vi "Read Actual Values.vi"(8 "Error In":errorcluster, 11 "INL DNL Test in":refnum<class "INL DNL Test.lvclass">) -> (0 "Error Out":errorcluster, 2 "Actual Values":T1, 3 "INL DNL Test out":refnum<class "INL DNL Test.lvclass">)   [LabVIEW 2020, in "INL DNL Test.lvclass"]
uses:
  INL DNL Test.lvclass
  Device/Parent/Typedef/Data Cluster.ctl
  INL DNL Test.lvclass/INL DNL Test.ctl
  Device/Parent/Device.lvclass
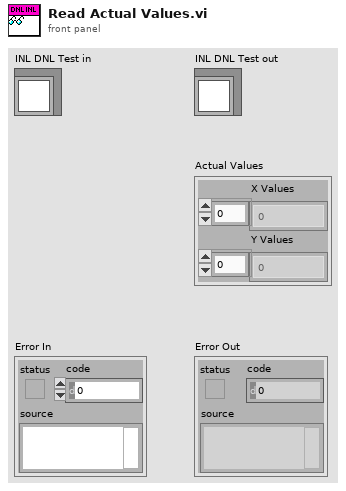
[diagram p1: front panel]
types:
  T1 = typedef "Device.lvclass/Data Cluster.ctl" = cluster{"X Values":dbl[], "Y Values":dbl[]}
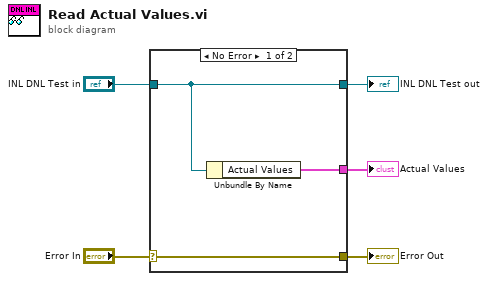
[diagram p0: block diagram]
diagram:
  n1 = case shown="No Error" "Error In" {
    selector: "Error In" -> [w8 w9]
    tunnel: [w8 w9] -> w4
    tunnel: [w7 w10] -> w2
    tunnel: "INL DNL Test in" -> [w7 w10]
    tunnel: [w6 _] -> w1
    frame No Error {
      n2 = Unbundle By Name(w7) -> ("Actual Values"=w6:T1)
    }
    frame Error {
    }
  }
  "Error Out" <- w4
  "INL DNL Test out" <- w2
  "Actual Values" <- w1
